vi "InitiateGeneration.vi"(8 "error in (no error)":errorcluster, 11 "IviFgen in":refnum<class "IviFgen.lvclass">) -> (0 "error out":errorcluster, 3 "IviFgen out":refnum<class "IviFgen.lvclass">)   [LabVIEW 2014, in "FgenPlugins.lvlib" / "IviFgen.lvclass"]
uses:
  IviFgen.lvclass
  FgenPluginBaseClass/FgenPluginsBase.lvclass/FgenPluginsBase.ctl
  FgenPluginBaseClass/Accessors/Read Channels.vi
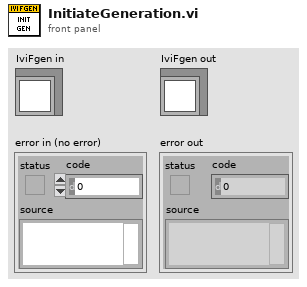
[diagram p1: front panel]
types:
  T1 = typedef "Channel.ctl" = cluster{"Name":string, "Enabled":bool, "Operation":enum16{"Continuous", "Burst"}, "Impedance (50)":dbl, "Handle":string, "Connected":bool, "Mode (Function)":enum16{"Function", "Arbitrary", "Sequence"}}
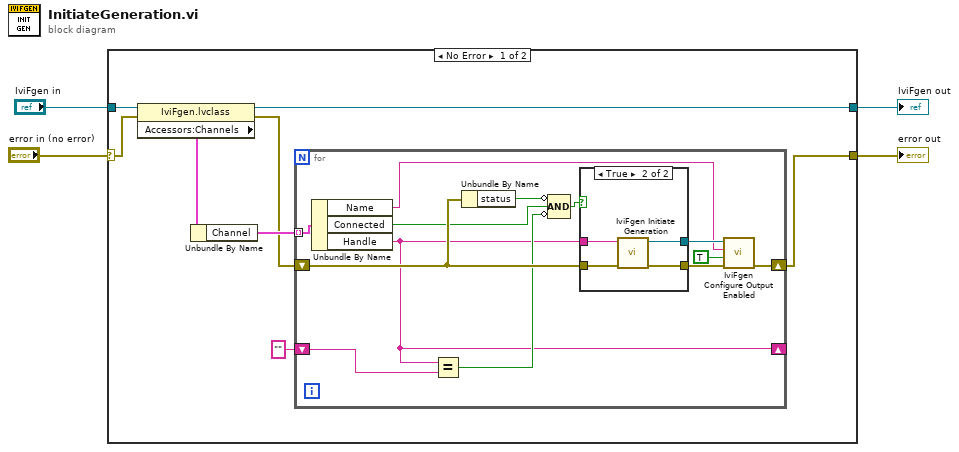
[diagram p0: block diagram]
diagram:
  n1 = case shown="No Error" "error in (no error)" {
    selector: "error in (no error)" -> [w11 w33]
    tunnel: "IviFgen in" -> [w12 w32]
    tunnel: [w5 w33] -> w2
    tunnel: [w6 w32] -> w1
    frame No Error {
      n2 = property class="IviFgen.lvclass"(reference=w12, error in=w11) -> (reference out=w6:refnum<class "IviFgen.lvclass">, error out=w8:errorcluster, "Accessors:Channels"=w10:cluster{"Count":u16, "Channel":T1[]})
      n3 = Unbundle By Name(w10) -> ("Channel"=w9:T1[])
      n4 = for {
        tunnel: w9 -> [w25] mode=indexing
        shift-right: [w18] -> _
        shift-left: "" ("Handle") -> [w24]
        shift-right: [w13] -> w5
        shift-left: w8 -> [w22]
        n5 = Unbundle By Name(w25) -> ("Name"=w15:string, "Connected"=w21:bool, "Handle"=w18:string)
        n6 = Equal?(x=w18, y=w24) -> (x = y?=w20:bool)
        n7 = Unbundle By Name(w22) -> ("status"=w19:bool)
        n8 = Compound Arithmetic op=AND(invert w19, w21, invert w20) -> (w23:bool)
        n9 = case shown="True" w23 {
          tunnel: w22 -> [w27 w31]
          tunnel: [w27 w30] -> w17
          tunnel: [w26 w29] -> w16
          tunnel: w18 -> [w26 w28]
          frame False {
          }
          frame True {
            n10 = call <vilib>:"IviFgen Initiate Generation.vi"("error in (no error)"=w31, "instrument handle"=w28) -> ("error out"=w30:errorcluster, "instrument handle out"=w29:refnum<k15>)  [unwired: 8 in]
          }
        }
        n11 = call <vilib>:"IviFgen Configure Output Enabled.vi"("error in (no error)"=w17, "channel enabled (True)"=TRUE, "channel name (\"CHANNEL1\")"=w15, "instrument handle"=w16) -> ("error out"=w13:errorcluster)  [unwired: 6 in, 1 out]
      }
    }
    frame Error {
    }
  }
  "error out" <- w2
  "IviFgen out" <- w1
